vi "getCamerasPositionByID.vi"(11 "Field Size 2":T1) -> (3 "Cameras Positions":dbl[][](array[numeric]))   [LabVIEW 2018]
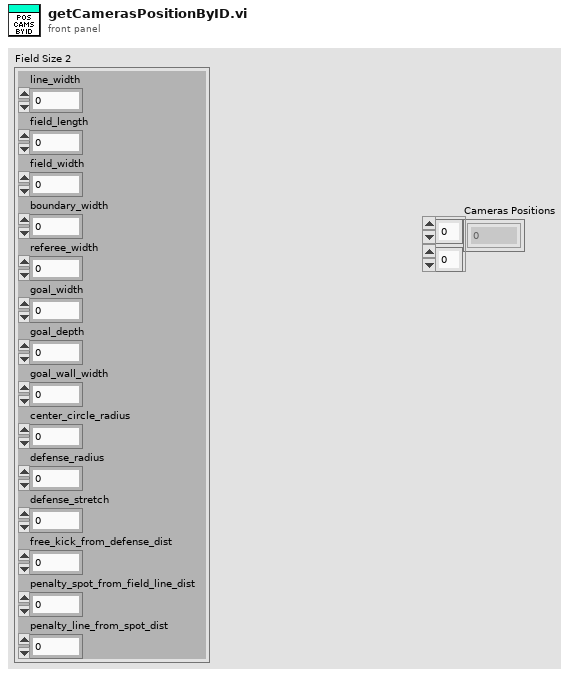
[diagram p1: front panel]
types:
  T1 = cluster{"line_width":u32, "field_length":u32, "field_width":u32, "boundary_width":u32, "referee_width":u32, "goal_width":u32, "goal_depth":u32, "goal_wall_width":u32, "center_circle_radius":u32, "defense_radius":u32, "defense_stretch":u32, "free_kick_from_defense_dist":u32, "penalty_spot_from_field_line_dist":u32, "penalty_line_from_spot_dist":u32}
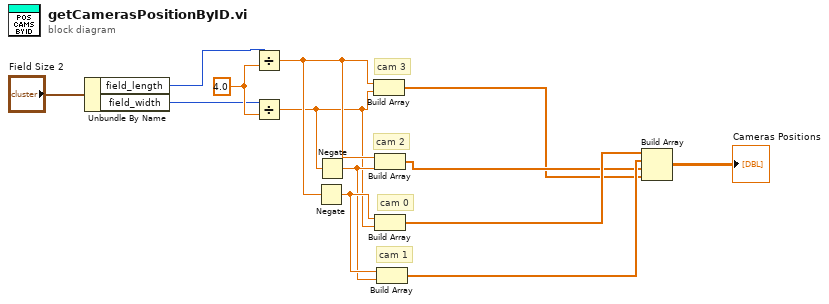
[diagram p0: block diagram]
diagram:
  w12 = 4.0 ("y")
  # "cam 1"
  # "cam 0"
  # "cam 2"
  # "cam 3"
  n1 = Unbundle By Name("Field Size 2") -> ("field_length"=w11:u32, "field_width"=w10:u32)
  n2 = Divide(x=w11, y=w12) -> (x/y=w8:dbl)
  n3 = Divide(x=w10, y=w12) -> (x/y=w6:dbl)
  n4 = Negate(x=w8) -> (-x=w9:dbl)
  n5 = Negate(x=w6) -> (-x=w7:dbl)
  n6 = Build Array(w8, w6) -> (w2:dbl[])
  n7 = Build Array(w8, w7) -> (w3:dbl[])
  n8 = Build Array(w9, w6) -> (w5:dbl[])
  n9 = Build Array(w9, w7) -> (w4:dbl[])
  n10 = Build Array(w5, w4, w3, w2) -> (→"Cameras Positions":dbl[][])
